vi "RandomFeed.vi"(8 "error in (no error)":errorcluster, 10 "Snake":refnum<class "Snake.lvclass">, 11 "Feeder in":refnum<class "Feeder.lvclass">) -> (0 "error out":errorcluster, 2 "FeedPos":T1, 3 "Feeder out":refnum<class "Feeder.lvclass">)   [LabVIEW 2018, in "Feeder.lvclass"]
uses:
  Feeder.lvclass
  Snake/Snake.lvclass
  Typedefs/XYposition.ctl
  Feeder.lvclass/Feeder.ctl
panel:
  # "Connector Pane"
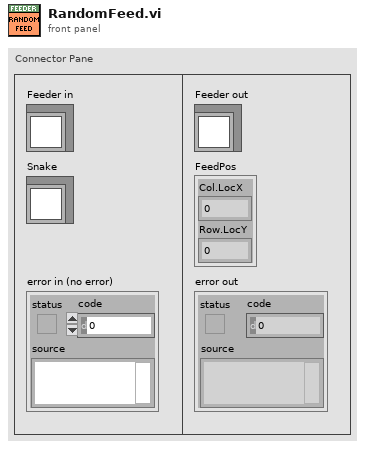
[diagram p1: front panel]
types:
  T1 = typedef "XYposition.ctl" = cluster{"Col.LocX":i32, "Row.LocY":i32}
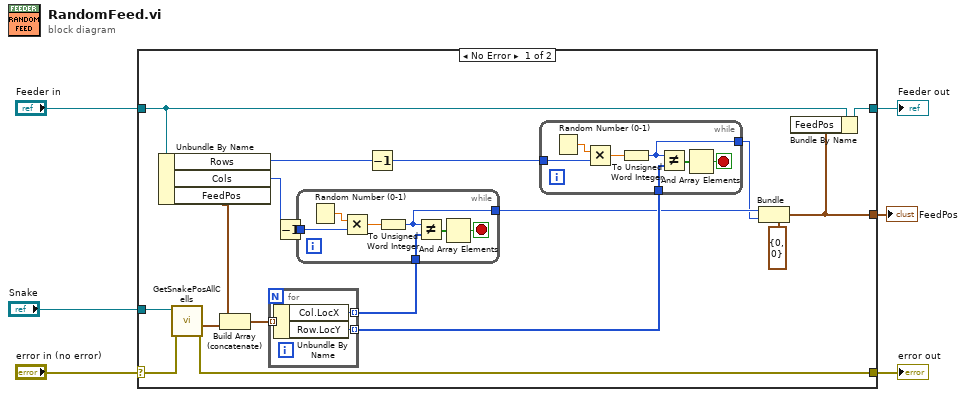
[diagram p0: block diagram]
diagram:
  n1 = case shown="No Error" "error in (no error)" {
    selector: "error in (no error)" -> [w23 w43]
    tunnel: [w22 w43] -> w5
    tunnel: [w10 w42] -> w3
    tunnel: "Feeder in" -> [w21 w42]
    tunnel: "Snake" -> [w24 _]
    tunnel: [w9 _] -> w1
    frame No Error {
      n2 = Unbundle By Name(w21) -> ("Rows"=w20:i32, "Cols"=w14:i32, "FeedPos"=w16:T1)
      n3 = call "GetSnakePosAllCells.vi"("error in (no error)"=w23, "Snake in"=w24) -> ("error out"=w22:errorcluster, "CellPositions"=w19:T1[])  [unwired: 6 in, 2 out]
      n4 = Build Array (concatenate)(w16, w19) -> (w17:T1[])
      n5 = for {
        tunnel: w17 -> [w41] mode=indexing
        tunnel: [w40] -> w15 mode=indexing
        tunnel: [w39] -> w18 mode=indexing
        n6 = Unbundle By Name(w41) -> ("Col.LocX"=w40:i32, "Row.LocY"=w39:i32)
      }
      n7 = Decrement(x=w14) -> (x-1=w8:i32)
      n8 = while {
        tunnel: w8 -> [w30]
        tunnel: w15 -> [w28]
        tunnel: [w25] -> w12
        stop <- w26 stop-if-true
        n9 = Random Number (0-1)() -> (number: 0 to 1=w31:dbl)
        n10 = Multiply(x=w31, y=w30) -> (x*y=w29:dbl)
        n11 = To Unsigned Word Integer(number=w29) -> (unsigned 16bit integer=w25:u16)
        n12 = Not Equal?(x=w25, y=w28) -> (x != y?=w27:bool[])
        n13 = And Array Elements(Boolean array=w27) -> (logical AND=w26:bool)
      }
      n14 = Decrement(x=w20) -> (x-1=w7:i32)
      n15 = while {
        tunnel: w7 -> [w37]
        tunnel: w18 -> [w35]
        tunnel: [w32] -> w11
        stop <- w33 stop-if-true
        n16 = Random Number (0-1)() -> (number: 0 to 1=w38:dbl)
        n17 = Multiply(x=w38, y=w37) -> (x*y=w36:dbl)
        n18 = To Unsigned Word Integer(number=w36) -> (unsigned 16bit integer=w32:u16)
        n19 = Not Equal?(x=w32, y=w35) -> (x != y?=w34:bool[])
        n20 = And Array Elements(Boolean array=w34) -> (logical AND=w33:bool)
      }
      n21 = Bundle(cluster=T1 {"Col.LocX"=0, "Row.LocY"=0} ("FeedPos"), "Col.LocX"=w12, "Row.LocY"=w11) -> (w9:T1)
      n22 = Bundle By Name(cluster=w21, "FeedPos"=w9) -> (w10:refnum<class "Feeder.lvclass">)
    }
    frame Error {
    }
  }
  "error out" <- w5
  "Feeder out" <- w3
  "FeedPos" <- w1
